vi "Fetch Multi Eval Meas ACLR EN-DC Results.vi"(8 "error in (no error)":errorcluster, 9 "Result Type (Current)":i32(ring) items=["Current", "Average"], 10 "Instance (1)":T2=1, 11 "VISA resource name":refnum<visa-resource-name>) -> (0 "error out":errorcluster, 1 "ACLR EN-DC Results":T1 {"EN-DC Positive" format="%^.3e"; "Carrier" format="%^.3e"; "EN-DC Negative" format="%^.3e"}, 2 "Reliability":i32, 3 "VISA resource name out":refnum<visa-resource-name>)   [LabVIEW 2020, in "Rohde&Schwarz CMWXP NR FR1 Measurement.lvlib"]
doc: "Returns the relative ACLR values for EN-DC, as displayed in the table below the ACLR diagram. The current and average values can be retrieved.\n\nAttributes:\nRSCMWXPNRFR1M_ATTR_FETCH_MULTI_EVAL_MEAS_ACLR_ENDC_CURRENT_RESULTS\nRSCMWXPNRFR1M_ATTR_FETCH_MULTI_EVAL_MEAS_ACLR_ENDC_AVERAGE_RESULTS\n\nRemote-control commands:\nFETCh:NRSub:MEAS<i>:MEValuation:ACLR:ENDC:CURRent?\nFETCh:NRSub:MEAS<i>:MEValuation:ACLR:ENDC:AVERage?"
uses:
  <instrlib>/Rohde&Schwarz CMWXP NR FR1 Measurement/Rohde&Schwarz CMWXP NR FR1 Measurement.lvlib
  <instrlib>/Rohde&Schwarz CMWXP NR FR1 Measurement/Private/_Instance.ctl
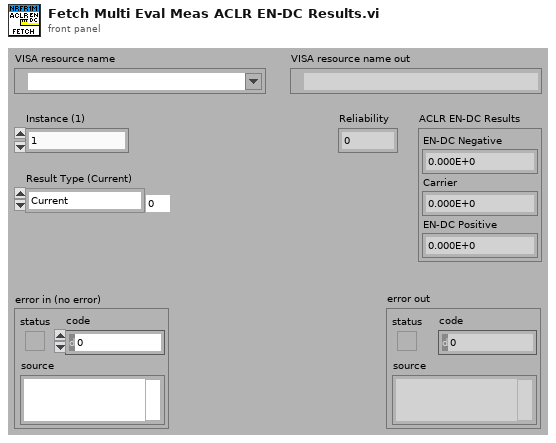
[diagram p1: front panel]
types:
  T1 = cluster{"EN-DC Negative":dbl, "Carrier":dbl, "EN-DC Positive":dbl}
  T2 = typedef "Rohde&Schwarz CMWXP NR FR1 Measurement.lvlib/_Instance.ctl" = i32
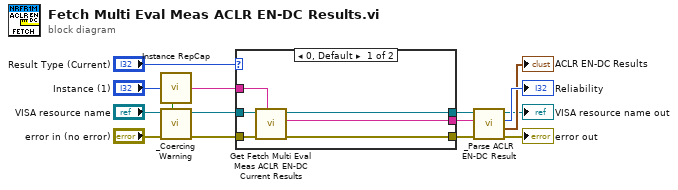
[diagram p0: block diagram]
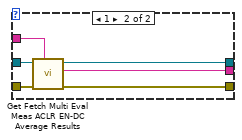
[diagram p2: hidden frame]
diagram:
  n1 = call <instrlib>:"Instance RepCap.vi"("Instance In"="Instance (1)") -> ("In Range?"=w12:bool, "RepCap Identifier Out"=w11:string)  [unwired: 1 in]
  n2 = call <instrlib>:"_Coercing Warning.vi"("In Range?"=w12, "error in (no error)"="error in (no error)", "VISA resource name"="VISA resource name") -> ("error out"=w9:errorcluster, "VISA resource name out"=w10:refnum<visa-resource-name>)  [unwired: 7 in]
  n3 = case shown="0, Default" "Result Type (Current)" {
    tunnel: w11 -> [w21 w27]
    tunnel: w10 -> [w20 w26]
    tunnel: w9 -> [w19 w25]
    tunnel: [w18 w24] -> w7
    tunnel: [w17 w23] -> w6
    tunnel: [w16 w22] -> w5
    frame 0, Default {
      n4 = call "Get Fetch Multi Eval Meas ACLR EN-DC Current Results"("Repeated Capabilities"=w21, "error in (no error)"=w19, "instrument handle"=w20) -> ("error out"=w18:errorcluster, "Fetch Multi Eval Meas ACLR EN-DC Current Results"=w17:string, "instrument handle out"=w16:refnum<visa-resource-name>)  [unwired: 6 in]
    }
    frame 1 {
      n5 = call "Get Fetch Multi Eval Meas ACLR EN-DC Average Results"("Repeated Capabilities"=w27, "error in (no error)"=w25, "instrument handle"=w26) -> ("error out"=w24:errorcluster, "Fetch Multi Eval Meas ACLR EN-DC Average Results"=w23:string, "instrument handle out"=w22:refnum<visa-resource-name>)  [unwired: 6 in]
    }
  }
  n6 = call <instrlib>:"_Parse ACLR EN-DC Result.vi"("error in (no error)"=w7, "Input String"=w6, "VISA resource name"=w5) -> ("error out"=→"error out":errorcluster, "ACLR EN-DC Results"=→"ACLR EN-DC Results":T1, "Reliability"=→"Reliability":i32, "VISA resource name out"=→"VISA resource name out":refnum<visa-resource-name>)  [unwired: 5 in]
